vi "Robot Global Data.vi"() -> ()   [LabVIEW 2018]
doc: "This global VI can contain as many global variables as you need. To create a global variable, place a control on the panel, give it a good name. To read or write to it from a VI, drag the icon to the diagram of that VI. You can also drag from the project. Click on the node to change which global you access. You shouldn't have multiple locations writing to a global or it will cause a race-condition."
uses:
  <vilib>/Rock Robotics/WPI/Camera/WPI_CameraImageSize.ctl
  <vilib>/Rock Robotics/WPI/DriverStation/WPI_DriverStationRobotMode2.ctl
panel:
  in  "Hatch Mover Scale":dbl=1.0 min=0.0 max=1.0 step=0.1
  in  "Elevator Scale":dbl=1.0 min=0.0 max=1.0 step=0.1
  in  "Autonomous Wait":u32=10
  in  "Climb Back Push Down":bool
  in  "Climb Back Push Up":bool
  in  "Hatch Mover Duration":dbl=5.0
  in  "Hatch Mover Setpoint":dbl=1.0
  in  "Climb Front Push Down":bool
  in  "Climb Front Push Up":bool
  in  "Hatch Mover Retract":bool
  in  "Hatch Mover Extend":bool
  in  "SlowModeSettings":i32=2
  in  "MaxSpeedSlow":dbl=0.4
  in  "SlowRate":dbl=1.0
  in  "MaxTurnSlow":dbl=0.55
  in  "MaxTurnRateSlow":dbl=20.0
  in  "Cargo Stop Current":dbl=10.0
  in  "Cargo Hold Duration":dbl=1.0
  out "Stop the grabber":bool
  in  "Cheezy Drive Mode":u32=2
  in  "Cargo Setpoint":dbl=1.0 min=0.0 max=1.0 step=0.1
  in  "Elevator Duration":dbl=2.0
  in  "Elevator Setpoint":dbl=1.0 min=0.0 max=1.0 step=0.1
  in  "Pivot Right Setpoint":dbl=0.3 min=0.0 max=1.0 step=0.1
  in  "Pivot Left Setpoint":dbl=0.3 min=0.0 max=1.0 step=0.1
  in  "Level Down":bool
  in  "Level Up":bool
  in  "Extention":dbl
  in  "Hatch Release":bool
  in  "Hatch Hold":bool
  in  "Cargo Release":bool
  in  "Cargo Hold":bool
  in  "Elevator":dbl
  in  "Right Pivot":bool
  in  "Left Pivot":bool
  in  "SlowMode":u32=2
  in  "Quickturn":bool
  in  "Select Mode":dbl
  in  "Speed":dbl
  in  "Turn":dbl
  in  "Robot Mode":T1=enum."Autonomous Enabled"
  in  "image size":T2=enum."320x240"
  in  "Enable Vision":bool=TRUE
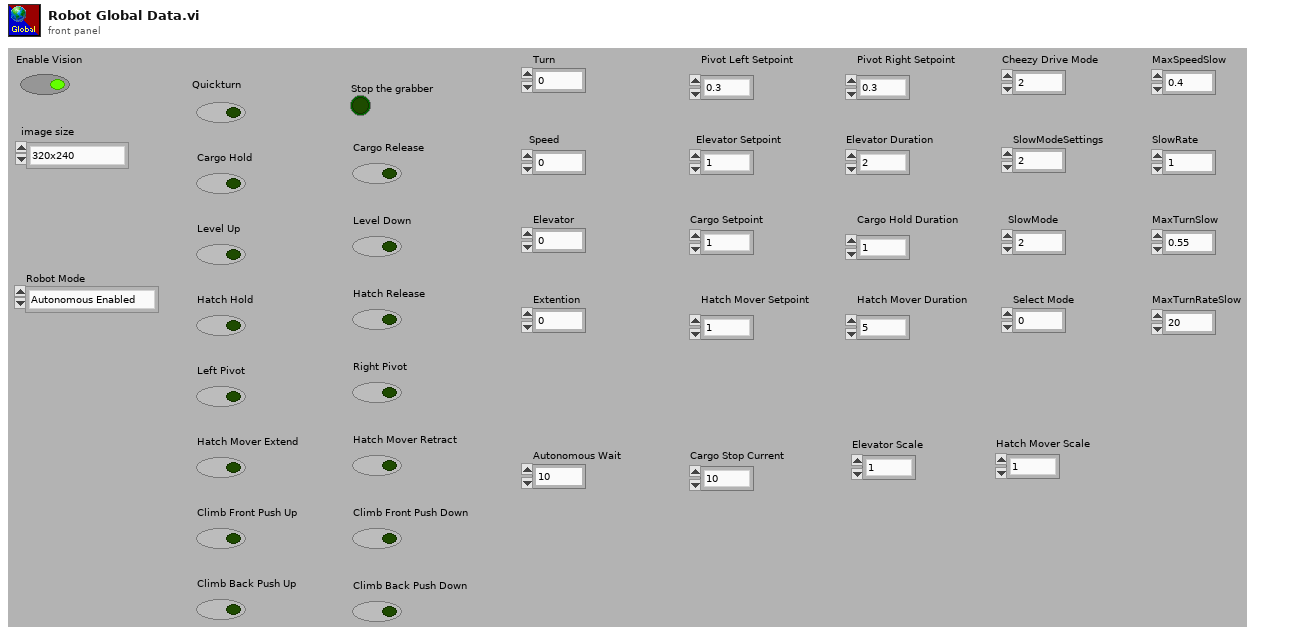
[diagram p1: front panel]
types:
  T1 = typedef "WPI_DriverStationRobotMode2.ctl" = enum16{"Autonomous Disabled", "Autonomous Enabled", "Teleop Disabled", "Teleop Enabled", "Disconnected", "Finish", "Test Disabled", "Test Enabled", "Emergency Stopped"}
  T2 = typedef "WPI_CameraImageSize.ctl" = enum16{"640x480", "320x240", "160x120", "Custom"}
diagram:
